vi "Excel Get Data (str).vi"(0 "report in":refnum<class "NI_report.lvclass">, 5 "data type":string, 7 "start (0, 0)":cluster{"start row":i32, "start column":i32}, 11 "error in (no error)":errorcluster, 12 "name (\"\")":string) -> (4 "report out":refnum<class "NI_report.lvclass">, 8 "data":string, 15 "error out":errorcluster)   [LabVIEW 2017, in "NI_Excel.lvclass"]
doc: "Retrieves data from the current worksheet. The data type you wire to the <B>data type</B> input determines the polymorphic instance to use."
uses:
  <vilib>/Utility/NIReport.llb/Excel/NI_Excel.lvclass
  <vilib>/Utility/NIReport.llb/NI_report.lvclass
  C:/Program Files (x86)/National Instruments/LabVIEW 2017/vi.lib/Utility/NIReport.llb/NI_report.lvclass
  <vilib>/Utility/NIReport.llb/Excel/NI_Excel.lvclass/NI_Excel.ctl
  <vilib>/addons/_office/NI_ReportGenerationToolkit.lvlib
  <vilib>/Utility/NIReport.llb/NI_ReportGenerationCore.lvlib
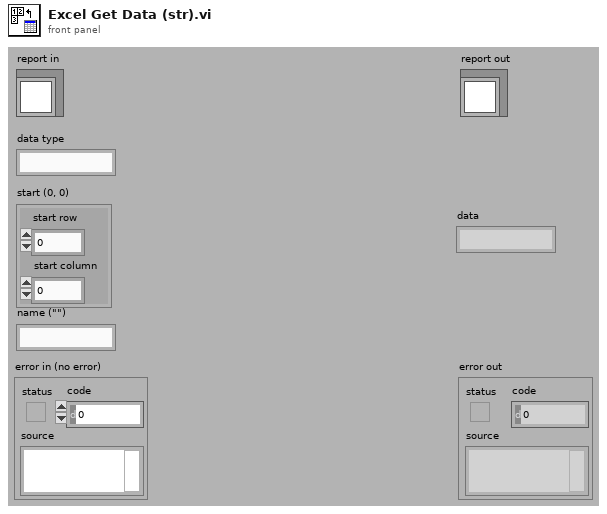
[diagram p1: front panel]
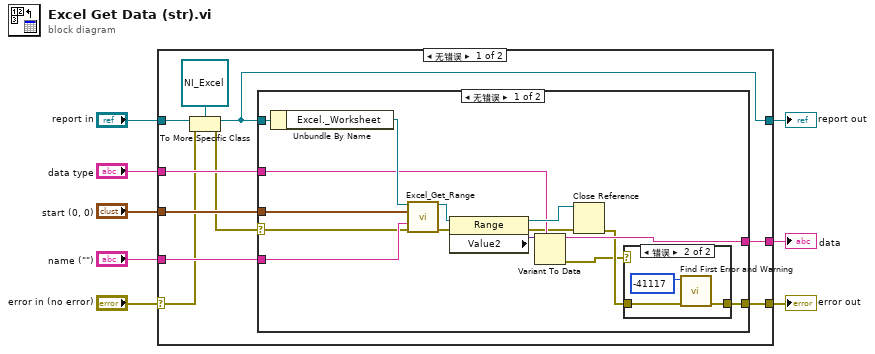
[diagram p0: block diagram]
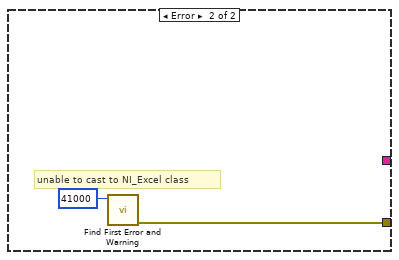
[diagram p3: hidden frame]
diagram:
  n1 = case shown="无错误" "error in (no error)" {
    selector: "error in (no error)" -> [w9 w41]
    tunnel: [w18 w41] -> w7
    tunnel: [w11 w40] -> w5
    tunnel: "report in" -> [w12 w40]
    tunnel: [w17 _] -> w4
    tunnel: "data type" -> [w16 _]
    tunnel: "start (0, 0)" -> [w15 _]
    tunnel: "name (\"\")" -> [w14 _]
    frame No Error {
      n2 = To More Specific Class(target class=refnum<class "NI_Excel.lvclass"> refnum ("report in"), reference=w12, error in=w9) -> (specific class reference=w11:refnum<class "NI_Excel.lvclass">, error out=w10:errorcluster)
      n3 = case shown="无错误" w10 {
        selector: w10 -> [w23 _]
        tunnel: [w22 w38] -> w18
        tunnel: [w29 _] -> w17
        tunnel: w16 -> [w27 _]
        tunnel: w15 -> [w26 _]
        tunnel: w14 -> [w25 _]
        tunnel: w11 -> [w24 _]
        frame No Error {
          n4 = Unbundle By Name(w24) -> ("Excel._Worksheet"=w28:refnum<k7>)
          n5 = call <vilib>:"Excel_Get_Range.vi"("Excel._Worksheet"=w28, "start"=w26, "name"=w25, "error in (no error)"=w23) -> ("Range"=w33:refnum<k7>, "error out"=w32:errorcluster)  [unwired: 1 in, 9 out]
          n6 = property class="Range"(reference=w33, error in=w32) -> (reference out=w31:refnum<k7>, error out=w19:errorcluster, "Value2"=w30:variant)
          n7 = Variant To Data(type=w27, Variant=w30) -> (data=w29:string, error out=w20:errorcluster)  [unwired: 1 in]
          n8 = Close Reference(reference=w31, error in (no error)=w19) -> (error out=w21:errorcluster)
          n9 = case shown="错误" w20 {
            tunnel: [w34 w36] -> w22
            tunnel: w21 -> [w34 w35]
            frame No Error {
            }
            frame Error {
              n10 = call <vilib>:"Find First Error and Warning.vi"("error in (no error)"=w35, "error code"=-41117) -> ("error out"=w36:errorcluster)  [unwired: 1 in, 4 out]
            }
          }
        }
        frame Error {
          # "unable to cast to NI_Excel class"
          n11 = call <vilib>:"Find First Error and Warning.vi"("error code"=41000) -> ("error out"=w38:errorcluster)  [unwired: 2 in, 4 out]
        }
      }
    }
    frame Error {
    }
  }
  "error out" <- w7
  "report out" <- w5
  "data" <- w4
